vi "StartAcquisition.vi"(8 "error in (no error)":errorcluster, 11 "reference in":refnum<class "Camera_Sim.lvclass">) -> (0 "error out":errorcluster, 3 "reference out":refnum<class "Camera_Sim.lvclass">)   [LabVIEW 2017, in "Camera_Sim.lvclass"]
doc: "Starts IMAQdx Acquisition. Use this with Grab."
uses:
  Camera_Sim.lvclass
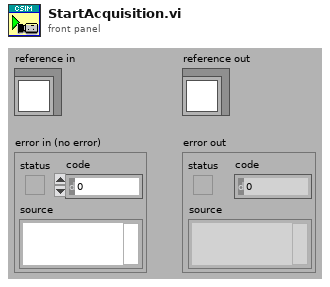
[diagram p1: front panel]
types:
  T1 = typedef "Image Type" = u32
  T2 = typedef "IMAQ Image.ctl" = refnum<image>
  T3 = typedef "CameraSim.lvclass/ObjectAttributes.ctl" = cluster{"Connected":bool, "Image Out":T2, "Frame Number":u32, "Path":path}
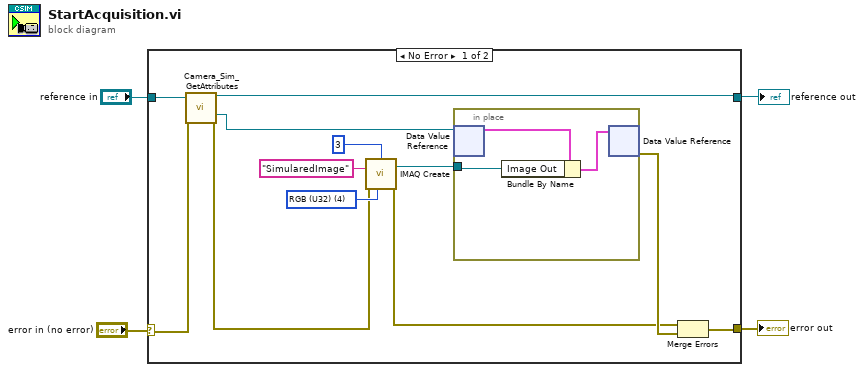
[diagram p0: block diagram]
diagram:
  n1 = case shown="No Error" "error in (no error)" {
    selector: "error in (no error)" -> [w15 w21]
    tunnel: [w13 w21] -> w3
    tunnel: [w11 w20] -> w1
    tunnel: "reference in" -> [w16 w20]
    frame No Error {
      w8 = T1 4 items=["Grayscale (U8)", "Grayscale (I16)", "Grayscale (SGL)", "Complex (CSG)", "RGB (U32)", "HSL (U32)", "RGB (U64)", "Grayscale (U16)"] ("Image Type")
      n2 = call "Camera_Sim_GetAttributes.vi"("reference in"=w16, "error in (no error)"=w15) -> ("reference out"=w11:refnum<class "Camera_Sim.lvclass">, "DataRef"=w12:refnum<data-value>, "error out"=w7:errorcluster)  [unwired: 10 in, 1 out]
      n3 = call "IMAQ Create"("Border Size"=3, "Image Name"="SimularedImage", "Image Type"=w8, "error in (no error)"=w7) -> ("New Image"=w5:T2, "error out"=w6:errorcluster)  [unwired: 1 out]
      n4 = in-place {
        in-place-border: w5 -> [w17]
        n5 = in-place-dvr #1(w12) -> (w19:T3)  [unwired: 1 out]
        n6 = Bundle By Name(cluster=w19, "Image Out"=w17) -> (w18:T3)
        n7 = in-place-dvr #1(w18) -> (w14:errorcluster)  [unwired: 1 out]
      }
      n8 = Merge Errors(w6, w14) -> (w13:errorcluster)
    }
    frame Error {
    }
  }
  "error out" <- w3
  "reference out" <- w1
